vi "Getlin.vi"(8 "error in (no error)":errorcluster, 11 "OneOfTemplate in":refnum<class "nixnet_grpc_FrameBufferResponse_frame.lvclass">) -> (0 "error out":errorcluster, 2 "Get_Val":T1, 3 "OneOfTemplate out":refnum<class "nixnet_grpc_FrameBufferResponse_frame.lvclass">)   [LabVIEW 2019, in "grpc-xnet_client.lvlib" / "nixnet_grpc_FrameBufferResponse_frame.lvclass"]
uses:
  nixnet_grpc_FrameBufferResponse_frame.lvclass
  nixnet_grpc_FrameResponse.ctl
  nixnet_grpc_FrameType.ctl
  nixnet_grpc_FrameFlags.ctl
  nixnet_grpc_FrameBufferResponse_frame.lvclass/nixnet_grpc_FrameBufferResponse_frame.ctl
  grpc-xnet_client.lvlib
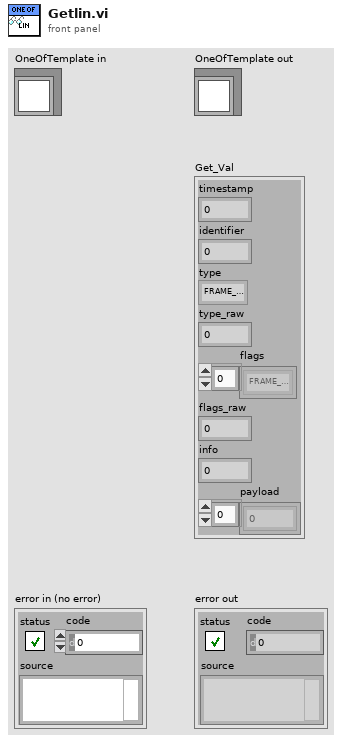
[diagram p1: front panel]
types:
  T1 = typedef "grpc-xnet_client.lvlib/nixnet_grpc_FrameResponse.ctl" = cluster{"timestamp":u64, "identifier":u32, "type":T2, "type_raw":u32, "flags":T3[], "flags_raw":u32, "info":u32, "payload":u8[]}
  T2 = typedef "grpc-xnet_client.lvlib/nixnet_grpc_FrameType.ctl" = enum32{"FRAME_TYPE_CAN_DATA", "FRAME_TYPE_CAN_REMOTE", "FRAME_TYPE_CAN_BUS_ERROR", "FRAME_TYPE_CAN20_DATA", "FRAME_TYPE_CANFD_DATA", "FRAME_TYPE_CANFDBRS_DATA", "FRAME_TYPE_FLEX_RAY_DATA", "FRAME_TYPE_FLEX_RAY_NULL", "FRAME_TYPE_FLEX_RAY_SYMBOL", "FRAME_TYPE_LIN_DATA", "FRAME_TYPE_LIN_BUS_ERROR", "FRAME_TYPE_LIN_NO_RESPONSE", "FRAME_TYPE_J1939_DATA", "FRAME_TYPE_SPECIAL_DELAY", "FRAME_TYPE_SPECIAL_LOG_TRIGGER", "FRAME_TYPE_SPECIAL_START_TRIGGER"}
  T3 = typedef "grpc-xnet_client.lvlib/nixnet_grpc_FrameFlags.ctl" = enum32{"FRAME_FLAGS_UNSPECIFIED", "FRAME_FLAGS_FLEX_RAY_STARTUP", "FRAME_FLAGS_FLEX_RAY_SYNC", "FRAME_FLAGS_FLEX_RAY_PREAMBLE", "FRAME_FLAGS_FLEX_RAY_CH_A", "FRAME_FLAGS_FLEX_RAY_CH_B", "FRAME_FLAGS_LIN_EVENT_SLOT", "FRAME_FLAGS_TRANSMIT_ECHO"}
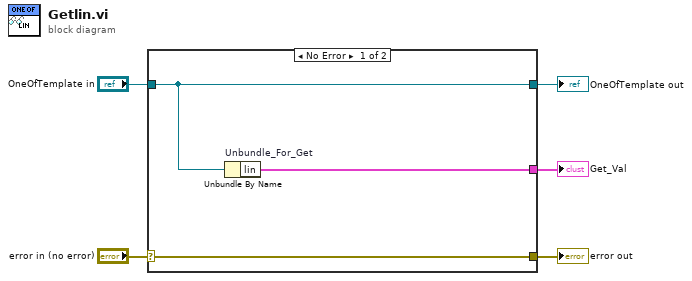
[diagram p0: block diagram]
diagram:
  n1 = case shown="No Error" "error in (no error)" {
    selector: "error in (no error)" -> [w8 w9]
    tunnel: [w8 w9] -> w4
    tunnel: [w7 w10] -> w2
    tunnel: "OneOfTemplate in" -> [w7 w10]
    tunnel: [w6 _] -> w1
    frame No Error {
      n2 = Unbundle By Name "Unbundle_For_Get"(w7) -> ("lin"=w6:T1)
    }
    frame Error {
    }
  }
  "error out" <- w4
  "OneOfTemplate out" <- w2
  "Get_Val" <- w1
